vi "复材超声C扫缺陷分析评定软件.vi"() -> ()   [LabVIEW 2018]
doc: "使用该模板构建用户界面事件处理设计模式。将模板应用于对话框及其它用户界面。用户也可创建并执行VI可按照与用户界面事件相同方式处理的用户定义事件。"
uses:
  <vilib>/Utility/NIReport.llb/Report Type.ctl
  <vilib>/addons/_office/_exclsub.llb/font.ctl
  <vilib>/Utility/NIReport.llb/HTML Report Image Alignment.ctl
  <vilib>/Utility/NIReport.llb/Append Report Text (str wrap).vi
  <vilib>/Utility/NIReport.llb/Append Image to Report (path wrap).vi
  <vilib>/addons/_office/word.llb/Word Easy Table (str).vi
  <vilib>/Utility/NIReport.llb/NI_report.lvclass
  <vilib>/vision/NI_Vision_Development_Module.lvlib
  <vilib>/Utility/NIReport.llb/Word/NI_Word.lvclass
  <vilib>/addons/_office/NI_ReportGenerationToolkit.lvlib
  <vilib>/Utility/NIReport.llb/NI_ReportGenerationCore.lvlib
panel:
  in  "删除标注":bool caption="定量分析"
  out "输入的灰度阈值":dbl caption="值"
  out "反射图原始路径":path
  out "穿透图原始路径":path
  out "ROImask":T1(plugin-control)
  in  "Operation 2":enum16{"overlay rectangle"}(ring)
  out "模式选择":u16(ring) items=["只读穿透图", "穿透图和反射图结合"]
  out "添加的路径":path
  out "连接的字符串 2":string
  out "临界面积百分比值":dbl
  out "临界Z值":i32
  out "标注后的图片路径":path
  out "弥散类检测结果合并":string[][](table)
  out "分层类检测结果合并":string[][](table)
  out "弥散类检测结果":string[][](table)
  out "分层类检测结果":string[][](table)
  out "部位信息":string[](array[string])=["", "34.500000", "32.500000", "1121", "34", "54.955926", "分层类", "不合格", ""]
  out "连接的字符串":string
  in  "完成标注":bool caption="定量分析"
  out "框数":dbl
  in  "Operation":enum16{"overlay rectangle"}(ring)
  out "自定义字体":T2={"Desired Font (Application)"=enum."Application Font", "[User-specified Font]"={"Font Name"="", "Size"=12, "Strikeout?"=FALSE, "Italic?"=FALSE, "Underline?"=FALSE, "Outline?"=FALSE, "Shadow?"=FALSE, "Bold?"=FALSE, "Rotation Angle"=0.0}, "Horizontal Alignment"=0, "Vertical Alignment"=0} {"Horizontal Alignment" items=["Left", "Center", "Right"]; "Vertical Alignment" items=["Bottom", "Top", "Baseline"]}
  out "框组":T3(array[cluster])
  out "质量等级":string
  out "灰度阈值":dbl
  in  "stop":bool caption="停止"
  in  "导入图像":bool caption="导入图片"
  in  "图像预处理":bool
  in  "自定义色彩":bool
  in  "开始标注":bool caption="定量分析"
  in  "查看标注":bool caption="辅助定性分析"
  in  "生成评定结果":bool caption="生成原始记录"
  in  "?":enum32{"穿透图", "反射图"}(tab)
  out "穿透图":T1(plugin-control)
  out "反射图":T1(plugin-control)
  out "产品规格":cluster{"产品长度（周长）（mm）":dbl, "产品宽度（母线长）（mm）":dbl}
  out "图像分辨率":T4
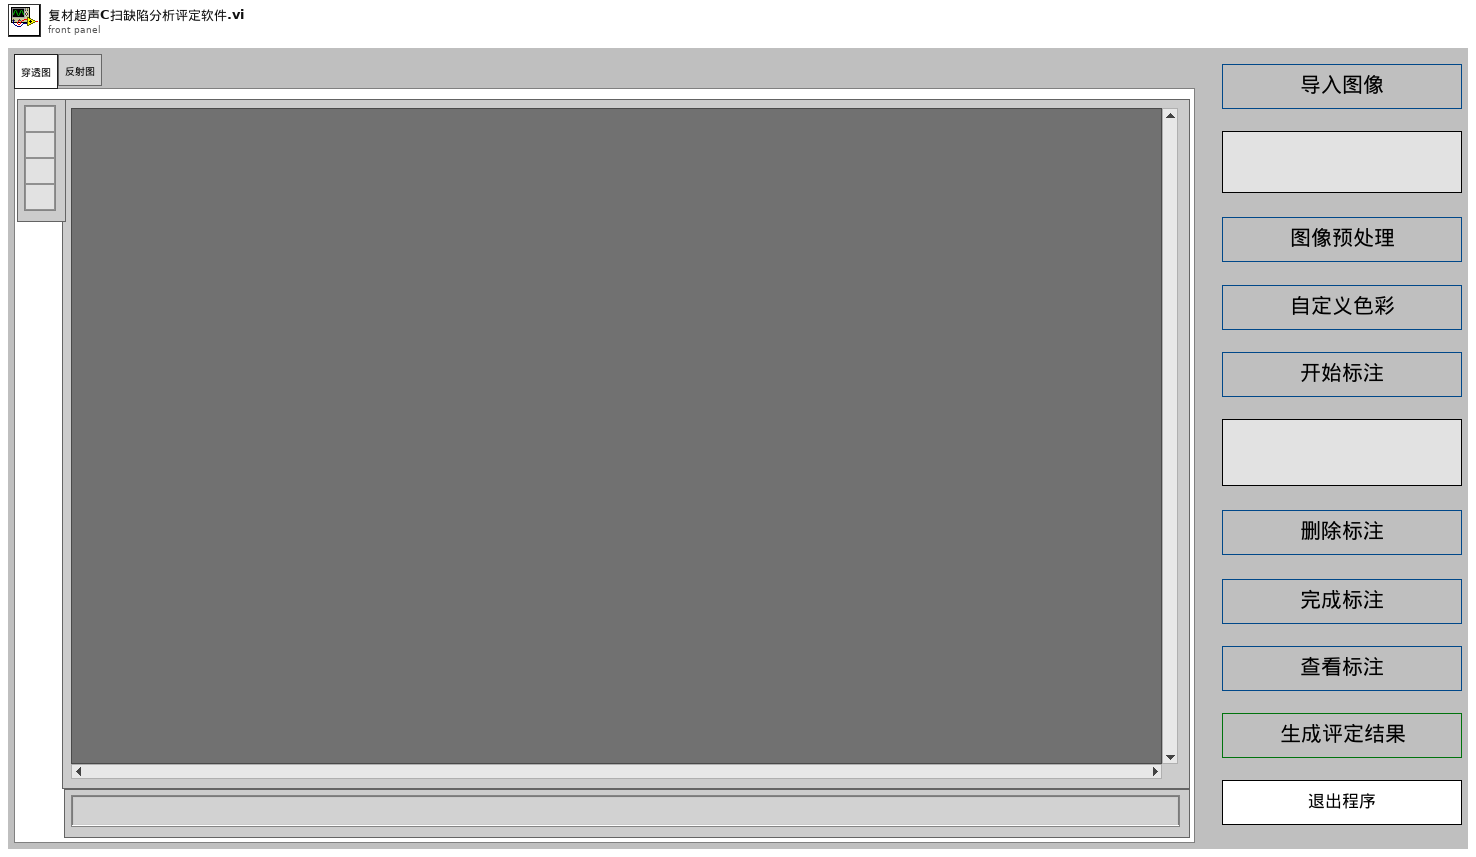
[diagram p1: front panel]
types:
  T1 = typedef "IMAQ Image.ctl" = refnum<image>
  T2 = cluster{"Desired Font (Application)":enum16{"User-specified Font", "Application Font", "System Font", "Dialog Font"}, "[User-specified Font]":cluster{"Font Name":string, "Size":i16, "Strikeout?":bool, "Italic?":bool, "Underline?":bool, "Outline?":bool, "Shadow?":bool, "Bold?":bool, "Rotation Angle":dbl}, "Horizontal Alignment":i16, "Vertical Alignment":i16}
  T3 = cluster{"Global Rectangle":i32[], "Contours":cluster{"Contour Type":u32, "ROI Type":u32, "Points":i32[]}[]}[]
  T4 = cluster{"图像X向分辨率（mm/像素）":dbl, "图像Y向分辨率（mm/像素）":dbl}
  T5 = cluster{"Zoom Tool":bool, "Selection Tool":bool, "Pan Tool":bool, "Point Tool":bool, "Line Tool":bool, "Rectangle Tool":bool, "Rotated Rectangle Tool":bool, "Polyline Tool":bool, "Polygon Tool":bool, "Freehand Tool":bool, "Closed Freehand Tool":bool, "Ellipse Tool":bool, "Annulus Tool":bool}
  T6 = enum32{"Invalid", "Standard", "Closed", "Hidden", "Minimized", "Maximized"}
  T7 = enum32{"Linear", "Log", "Exp", "Square", "Square root", "Power X", "Power 1/X"}
  T8 = enum32{"Gray", "Binary", "Gradient", "Rainbow", "Temperature"}
  T9 = enum16{"maximized", "minimized", "normal", "no change"}
  T10 = typedef "NI_ReportGenerationCore.lvlib/Report Type.ctl" = enum16{"HTML", "Word", "Excel"}
  T11 = typedef "NI_ReportGenerationCore.lvlib/HTML Report Image Alignment.ctl" = enum16{"(default)", "LEFT", "RIGHT", "TOP", "TEXTTOP", "MIDDLE", "ABSMIDDLE", "BASELINE", "BOTTOM", "ABSBOTTOM"}
  T12 = cluster{"position (Excel)":cluster{"row":i32, "column":i32}, "name (Excel)":string, "bookmark (Word)":string}
  T13 = cluster{"position (excel)":cluster{"row":i32, "column":i32}, "name (excel)":string, "bookmark (word)":string}
  T14 = typedef "NI_ReportGenerationToolkit.lvlib/font.ctl" = cluster{"font name":string, "font size":dbl, "bold":u16, "italic":u16, "underline":u16, "strike through":u16, "font color":u32}
  T15 = typedef "Image Type" = u32
  T16 = cluster{"Red (or Hue) value":u8, "Green (or Sat) value":u8, "Blue (or Light or Val) value":u8}[]
  T17 = cluster{"Global Rectangle":i32[], "Contours":cluster{"Contour Type":u32, "ROI Type":u32, "Points":i32[]}[]}
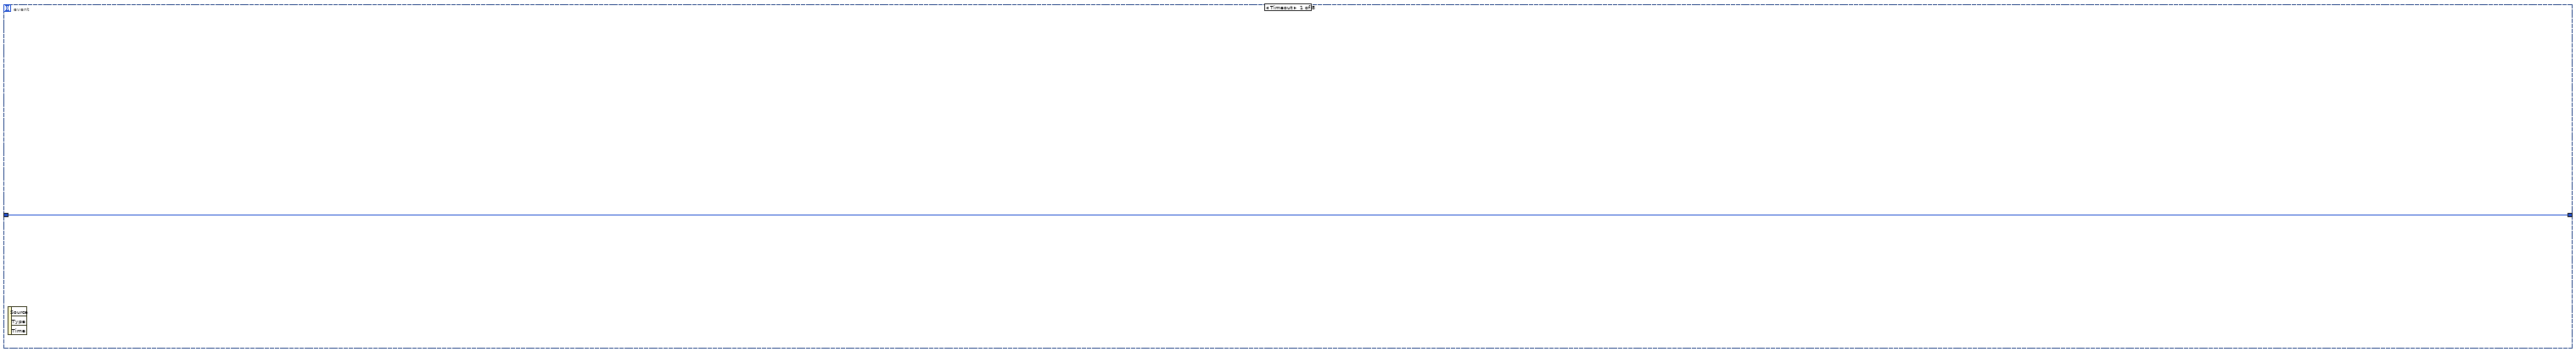
[diagram p3: hidden frame]
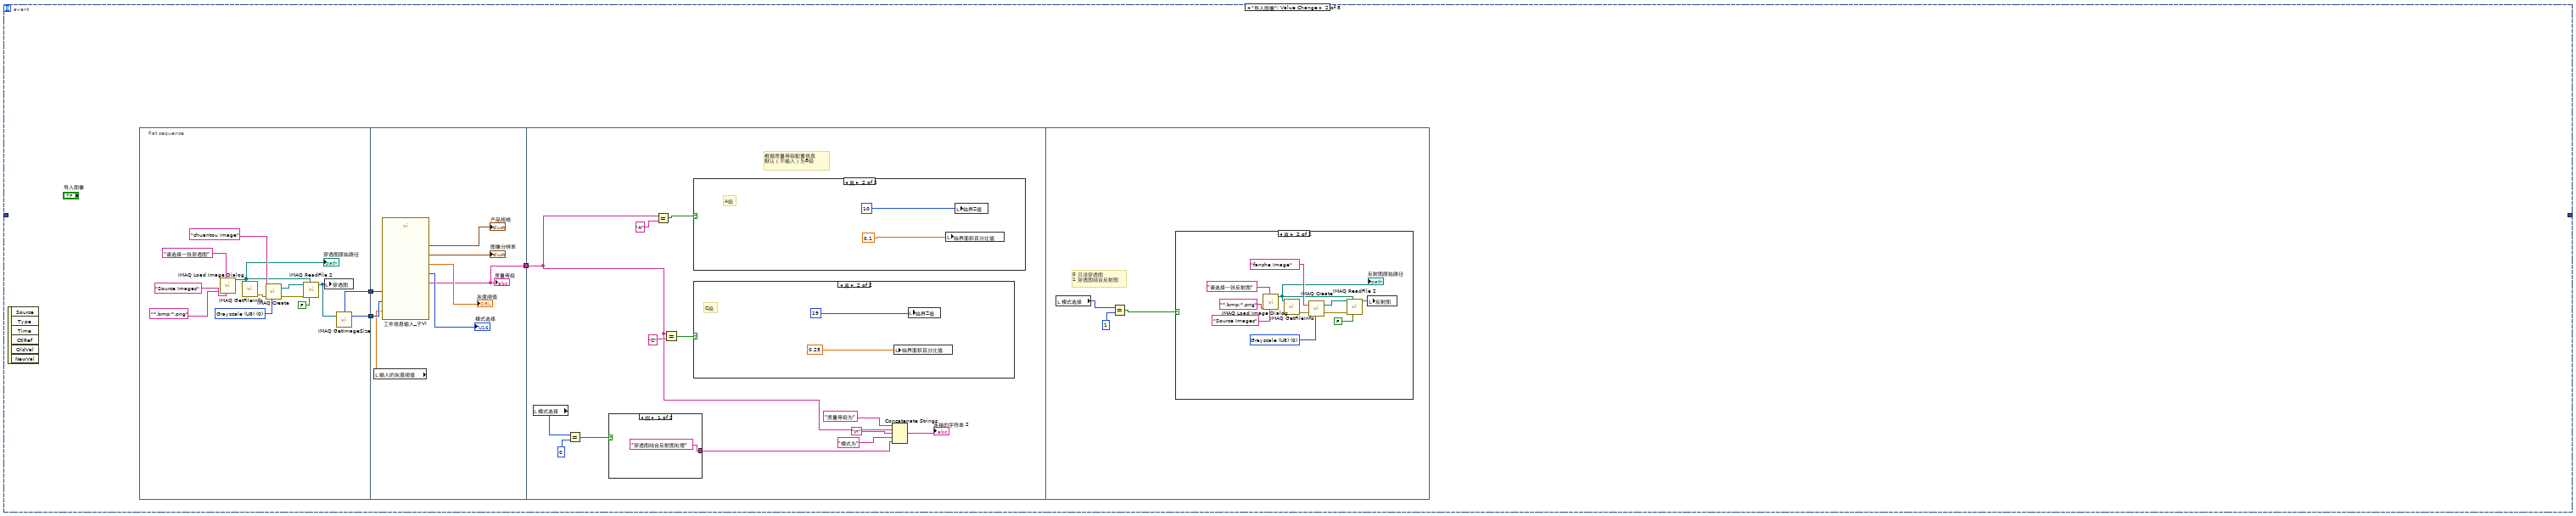
[diagram p4: hidden frame]
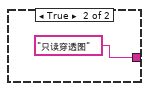
[diagram p5: hidden frame]
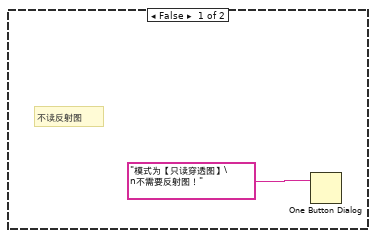
[diagram p8: hidden frame]
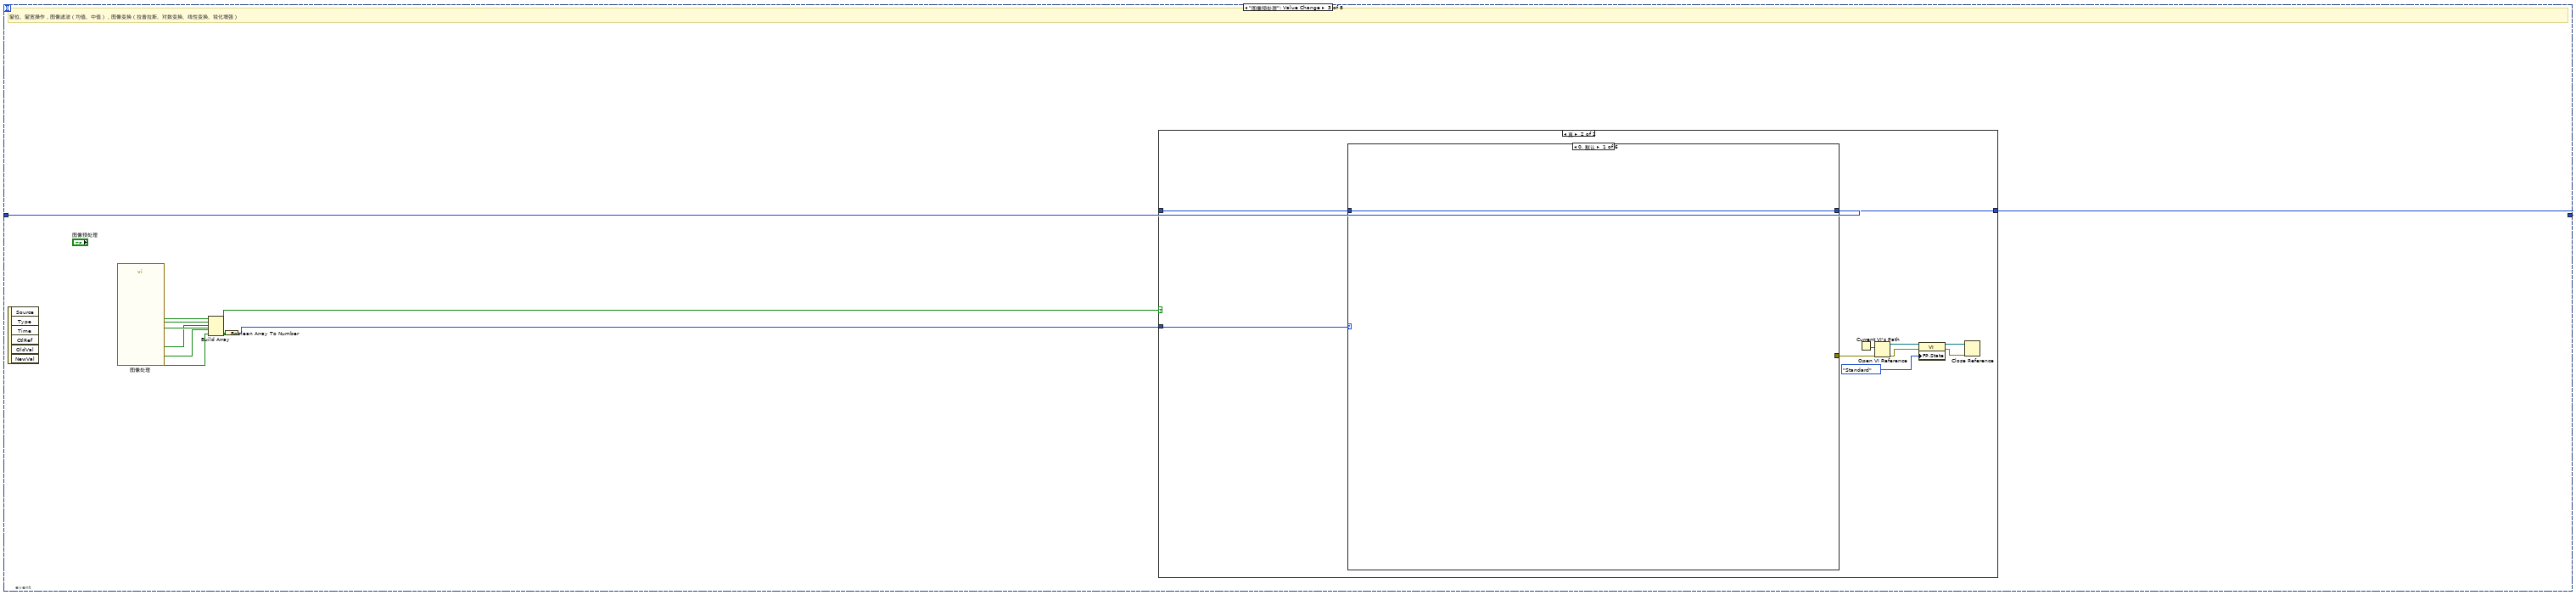
[diagram p9: hidden frame]
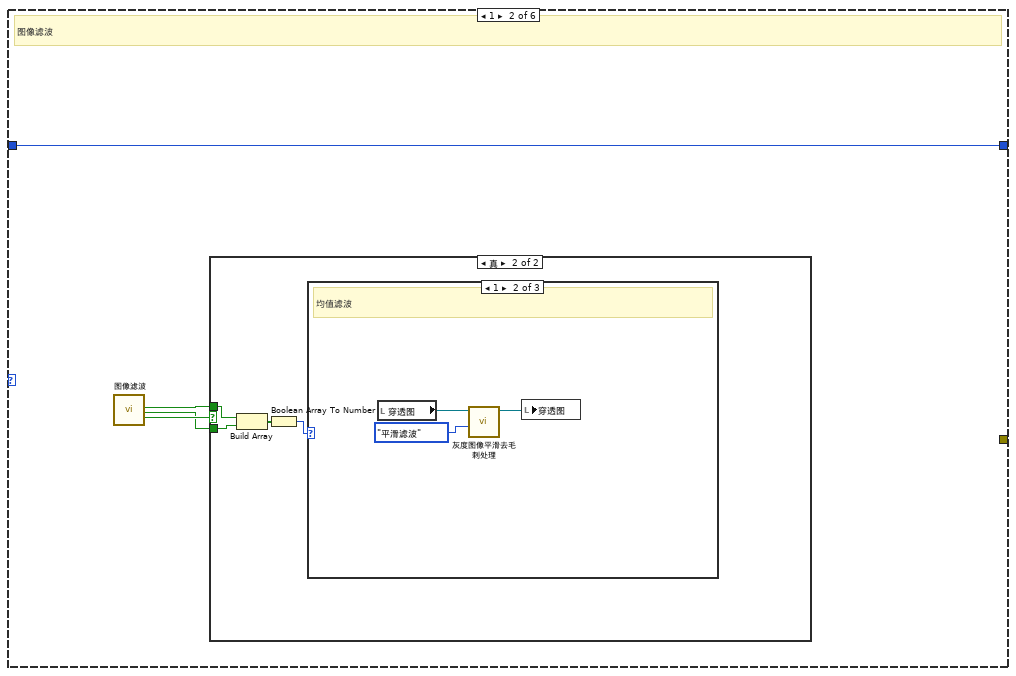
[diagram p11: hidden frame]
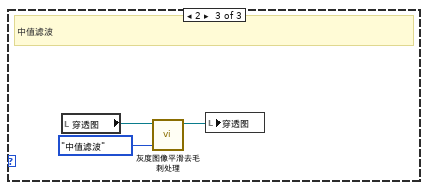
[diagram p14: hidden frame]
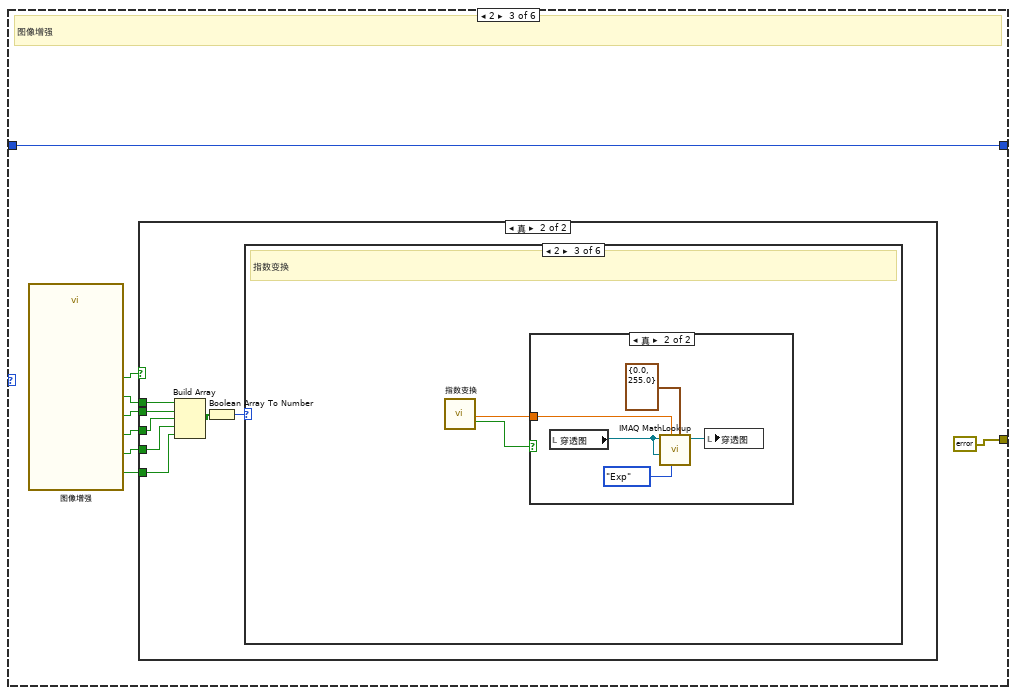
[diagram p15: hidden frame]
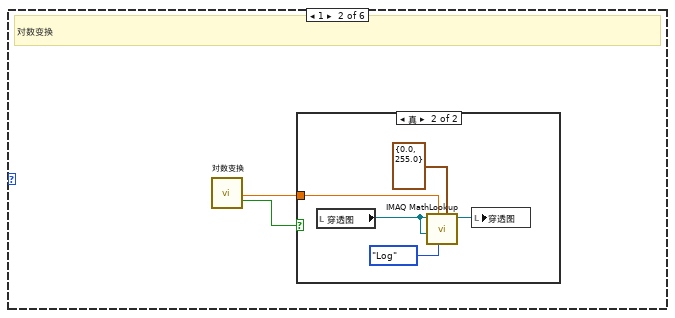
[diagram p18: hidden frame]
diagram:
  w12 = u16 0 items=["只读穿透图", "穿透图和反射图结合"] ("模式选择")
  w1 = FALSE ("查看标注")
  w17 = u32 0 items=["Grayscale", "Binary", "Gradient", "Rainbow", "Temperature", "User Defined", "Binary 16 Bit", "Gradient 16 Bit", "Rainbow 16 Bit", "Temperature 16 Bit", "User Defined 16 Bit"] ("Palette:Palette Type")
  w21 = TRUE ("Zoom to Fit Mode")
  w24 = u32 0 items=["Grayscale", "Binary", "Gradient", "Rainbow", "Temperature", "User Defined", "Binary 16 Bit", "Gradient 16 Bit", "Rainbow 16 Bit", "Temperature 16 Bit", "User Defined 16 Bit"] ("Palette:Palette Type")
  # "默认B级作为评判标准"
  n1 = flat-sequence {
    tunnel: [w28] -> w9
    tunnel: [w27] -> w8
    tunnel: [w26] -> w3
    tunnel: w9 -> [w31]
    tunnel: w8 -> [w32]
    tunnel: [w32] -> w7
    tunnel: [w31] -> w6
    tunnel: [w30] -> w4
    tunnel: w7 -> [w36]
    tunnel: w6 -> [w35]
    tunnel: [w34] -> w5
    frame #0 {
      w27 = "复材分析评定软件" ("section")
      w28 = "判定阈值配置" ("文件名称")
      n2 = call "ini配置文件读取（DBL）.vi"("key"="Z值", "section"=w27, "文件名称"=w28) -> ("value"=w26:dbl)  [unwired: 8 in]
    }
    frame #1 {
      n3 = call "ini配置文件读取（DBL）.vi"("key"="弥散性缺陷阈值", "section"=w32, "文件名称"=w31) -> ("value"=w30:dbl)  [unwired: 8 in]
    }
    frame #2 {
      n4 = call "ini配置文件读取（DBL）.vi"("key"="灰度阈值", "section"=w36, "文件名称"=w35) -> ("value"=w34:dbl)  [unwired: 8 in]
    }
  }
  n5 = To Long Integer(number=w3) -> (32bit integer=→"临界Z值":i32)
  n6 = property on="穿透图" class="ImageControl"("Palette Type"=w24, "ROI Tool Buttons Visible"=T5 {"Zoom Tool"=TRUE, "Selection Tool"=TRUE, "Pan Tool"=TRUE, "Point Tool"=FALSE, "Line Tool"=FALSE, "Rectangle Tool"=TRUE, "Rotated Rectangle Tool"=FALSE, "Polyline Tool"=FALSE, "Polygon Tool"=FALSE, "Freehand Tool"=FALSE, "Closed Freehand Tool"=FALSE, "Ellipse Tool"=FALSE, "Annulus Tool"=FALSE} ("ROI Tool Buttons Visible:All Elements")) -> ()  [unwired: 2 in, 2 out]
  n7 = property on="反射图" class="ImageControl"("Palette Type"=w17, "ROI Tool Buttons Visible"=T5 {"Zoom Tool"=TRUE, "Selection Tool"=TRUE, "Pan Tool"=TRUE, "Point Tool"=FALSE, "Line Tool"=FALSE, "Rectangle Tool"=TRUE, "Rotated Rectangle Tool"=FALSE, "Polyline Tool"=FALSE, "Polygon Tool"=FALSE, "Freehand Tool"=FALSE, "Closed Freehand Tool"=FALSE, "Ellipse Tool"=FALSE, "Annulus Tool"=FALSE} ("ROI Tool Buttons Visible:All Elements")) -> ()  [unwired: 2 in, 2 out]
  n8 = local write "标注后的图片路径"(path "" ("标注后的图片路径")) -> ()
  n9 = local write "连接的字符串 2"("（配置信息）" ("连接的字符串 2")) -> ()
  n10 = local write "连接的字符串"("（标注信息）" ("连接的字符串")) -> ()
  n11 = property on="穿透图" class="ImageControl"("Zoom to Fit Mode"=w21) -> ()  [unwired: 2 in, 2 out]
  n12 = property on="反射图" class="ImageControl"("Zoom to Fit Mode"=w21) -> ()  [unwired: 2 in, 2 out]
  n13 = local write "删除标注"(w1) -> ()
  n14 = local write "查看标注"(w1) -> ()
  n15 = local write "模式选择"(w12) -> ()
  n16 = local write "stop"(w1) -> ()
  n17 = local write "完成标注"(w1) -> ()
  n18 = while {
    shift-right: [w38] -> _
    shift-left: 0 -> [w39]
    stop <- w41 stop-if-true
    n19 = event shown="[4] \"开始标注\": 鼠标按下" {
      selector: _ -> [_ _ _ _ _ _ _ _]
      dyn-events: _ -> [_ _ _ _ _ _ _ _]
      timeout: 100 -> [_ _ _ _ _ _ _ _]
      tunnel: [_ _ _ _ _ _ _ w756] -> w41
      tunnel: w39 -> [w42 _ w102 w240 _ _ w595 _]
      tunnel: [w42 _ w101 w240 _ _ w595 0] -> w38
      event Timeout {
        n20 = event-data() -> ()  [unwired: 1 in, 3 out]
      }
      event "导入图像": Value Change {
        n21 = event-data() -> ()  [unwired: 1 in, 6 out]
        n22 = flat-sequence {
          tunnel: [w47] -> w44
          tunnel: [w46] -> w43
          tunnel: [w62] -> w45
          tunnel: w44 -> [w61]
          tunnel: w43 -> [w60]
          tunnel: w45 -> [w71]
          frame #0 {
            w50 = T15 0 items=["Grayscale (U8)", "Grayscale (I16)", "Grayscale (SGL)", "Complex (CSG)", "RGB (U32)", "HSL (U32)", "RGB (U64)", "Grayscale (U16)"] ("Image Type")
            n23 = call "IMAQ Load Image Dialog"("Pattern Label"="Source Images", "Prompt"="请选择一张穿透图" ("prompt"), "Pattern"="*.bmp;*.png") -> ("Path"=w49:path)  [unwired: 6 in, 2 out]
            "穿透图原始路径" <- w49
            n24 = call "IMAQ GetFileInfo"("File Path"=w49) -> ("error out"=w53:errorcluster)  [unwired: 4 in, 6 out]
            n25 = call "IMAQ Create"("Image Name"="chuantou Image", "Image Type"=w50, "error in (no error)"=w53) -> ("New Image"=w54:T1, "error out"=w55:errorcluster)  [unwired: 2 in]
            n26 = call "IMAQ ReadFile 2"("Use File Path Image Type"=FALSE, "File Path"=w49, "error in (no error)"=w55, "Image"=w54) -> ("Image Out"=w48:T1)  [unwired: 3 in, 4 out]
            n27 = local write "穿透图"(w48) -> ()
            n28 = call "IMAQ GetImageSize"("Image"=w48) -> ("Y Resolution"=w46:i32, "X Resolution"=w47:i32)  [unwired: 3 in, 1 out]
          }
          frame #1 {
            n29 = local read "输入的灰度阈值"() -> (w59:dbl)
            n30 = call "工件信息输入_子VI.vi"("Y Resolution"=w60, "X Resolution"=w61, "输入的灰度阈值"=w59) -> ("质量等级"=w62:string, "模式选择"=→"模式选择":u16, "灰度阈值"=→"灰度阈值":dbl, "产品规格"=→"产品规格":cluster{"产品长度（周长）（mm）":dbl, "产品宽度（母线长）（mm）":dbl}, "图像分辨率"=→"图像分辨率":T4)  [unwired: 3 in]
            "质量等级" <- w62
          }
          frame #2 {
            # "根据质量等级配置信息\n默认（不输入）为B级"
            n31 = local read "模式选择"() -> (w69:u16)
            n32 = Equal?(x=w69, y=u16 0) -> (x = y?=w68:bool)
            n33 = case shown="假" w68 {
              tunnel: ["穿透图结合反射图处理" ("字符串") "只读穿透图" ("字符串")] -> w67
              frame False {
              }
              frame True {
              }
            }
            n34 = Equal?(x=w71, y="A") -> (x = y?=w74:bool)
            n35 = Equal?(x=w71, y="C") -> (x = y?=w75:bool)
            n36 = case shown="真" w74 {
              frame False {
              }
              frame True {
                # "A级"
                n37 = local write "临界面积百分比值"(0.1 ("临界面积百分比值")) -> ()
                n38 = local write "临界Z值"(10 ("临界Z值")) -> ()
              }
            }
            n39 = case shown="真" w75 {
              frame False {
              }
              frame True {
                # "C级"
                n40 = local write "临界面积百分比值"(0.25 ("临界面积百分比值")) -> ()
                n41 = local write "临界Z值"(19 ("临界Z值")) -> ()
              }
            }
            n42 = Concatenate Strings("质量等级为" ("字符串"), w71, "\n", "模式为" ("字符串"), w67) -> (→"连接的字符串 2":string)
          }
          frame #3 {
            # "0 只读穿透图\n1 穿透图结合反射图"
            n43 = local read "模式选择"() -> (w87:u16)
            n44 = Equal?(x=w87, y=u16 1) -> (x = y?=w86:bool)
            n45 = case shown="真" w86 {
              frame False {
                # "不读反射图"
                n46 = One Button Dialog(message="模式为【只读穿透图】\n不需要反射图！" ("消息")) -> ()  [unwired: 1 in, 1 out]
              }
              frame True {
                w92 = T15 0 items=["Grayscale (U8)", "Grayscale (I16)", "Grayscale (SGL)", "Complex (CSG)", "RGB (U32)", "HSL (U32)", "RGB (U64)", "Grayscale (U16)"] ("Image Type")
                n47 = call "IMAQ Load Image Dialog"("Pattern Label"="Source Images", "Prompt"="请选择一张反射图" ("prompt"), "Pattern"="*.bmp;*.png") -> ("Path"=w91:path)  [unwired: 6 in, 2 out]
                "反射图原始路径" <- w91
                n48 = call "IMAQ GetFileInfo"("File Path"=w91) -> ("error out"=w95:errorcluster)  [unwired: 4 in, 6 out]
                n49 = call "IMAQ Create"("Image Name"="fanshe Image", "Image Type"=w92, "error in (no error)"=w95) -> ("New Image"=w96:T1, "error out"=w97:errorcluster)  [unwired: 2 in]
                n50 = call "IMAQ ReadFile 2"("Use File Path Image Type"=FALSE, "File Path"=w91, "error in (no error)"=w97, "Image"=w96) -> ("Image Out"=w90:T1)  [unwired: 3 in, 4 out]
                n51 = local write "反射图"(w90) -> ()
              }
            }
          }
        }
      }
      event "图像预处理": Value Change {
        # "窗位、窗宽操作，图像滤波（均值、中值），图像变换（拉普拉斯、对数变换、线性变换、锐化增强）"
        n52 = event-data() -> ()  [unwired: 1 in, 6 out]
        n53 = call "图像处理"() -> ("撤销图像处理"=w103:bool, "线性灰度值测量"=w104:bool, "窗位窗宽"=w109:bool, "图像增强"=w105:bool, "图像滤波"=w110:bool, "确定"=w106:bool)  [unwired: 13 in, 1 out]
        n54 = Build Array(w110, w105, w109, w104, w103) -> (w108:bool[])
        n55 = Boolean Array To Number(Boolean array=w108) -> (number=w107:u32)
        n56 = case shown="真" w106 {
          tunnel: w107 -> [_ w121]
          tunnel: w102 -> [w111 w113]
          tunnel: [w111 w112] -> w101
          frame False {
          }
          frame True {
            n57 = case shown="0, 默认" w121 {
              tunnel: [_ _ errorcluster {"status"=FALSE, "code"=0, "source"=""} ("错误输入（无错误）") _ _ _] -> w114
              tunnel: w113 -> [w122 w123 w137 w186 w209 w231]
              tunnel: [w122 w123 w137 w186 w209 w231] -> w112
              frame 0, Default {
              }
              frame 1 {
                # "图像滤波"
                n58 = call "图像滤波"() -> ("均值滤波"=w125:bool, "中值滤波"=w124:bool, "确定"=w126:bool)  [unwired: 16 in, 1 out]
                n59 = case shown="真" w126 {
                  tunnel: w125 -> [_ w129]
                  tunnel: w124 -> [_ w128]
                  frame False {
                  }
                  frame True {
                    n60 = Build Array(w129, w128) -> (w130:bool[])
                    n61 = Boolean Array To Number(Boolean array=w130) -> (number=w127:u32)
                    n62 = case shown="1" w127 {
                      frame 0, Default {
                      }
                      frame 1 {
                        # "均值滤波"
                        n63 = local read "穿透图"() -> (w133:T1)
                        n64 = call "灰度图像平滑去毛刺处理.vi"("滤波方法选择"=enum16{"中值滤波", "平滑滤波"}."平滑滤波", "Image"=w133) -> ("Image Out"=w132:T1)  [unwired: 9 in]
                        n65 = local write "穿透图"(w132) -> ()
                      }
                      frame 2 {
                        # "中值滤波"
                        n66 = local read "穿透图"() -> (w136:T1)
                        n67 = call "灰度图像平滑去毛刺处理.vi"("滤波方法选择"=enum16{"中值滤波", "平滑滤波"}."中值滤波", "Image"=w136) -> ("Image Out"=w135:T1)  [unwired: 9 in]
                        n68 = local write "穿透图"(w135) -> ()
                      }
                    }
                  }
                }
              }
              frame 2 {
                # "图像增强"
                n69 = call "图像增强"() -> ("幂变换"=w139:bool, "阈值变换"=w140:bool, "高斯变换"=w141:bool, "指数变换"=w142:bool, "对数变换"=w143:bool, "确定"=w144:bool)  [unwired: 13 in, 1 out]
                n70 = case shown="真" w144 {
                  tunnel: w143 -> [_ w149]
                  tunnel: w142 -> [_ w148]
                  tunnel: w141 -> [_ w147]
                  tunnel: w140 -> [_ w146]
                  tunnel: w139 -> [_ w145]
                  frame False {
                  }
                  frame True {
                    n71 = Build Array(w149, w148, w147, w146, w145) -> (w151:bool[])
                    n72 = Boolean Array To Number(Boolean array=w151) -> (number=w150:u32)
                    n73 = case shown="2" w150 {
                      frame 0, Default {
                      }
                      frame 1 {
                        # "对数变换"
                        n74 = call "对数变换"() -> ("变换系数K"=w152:dbl, "确定"=w153:bool)  [unwired: 17 in, 1 out]
                        n75 = case shown="真" w153 {
                          tunnel: w152 -> [_ w154]
                          frame False {
                          }
                          frame True {
                            n76 = local read "穿透图"() -> (w158:T1)
                            n77 = call "IMAQ MathLookup"("Range"=cluster{"Minimum":sgl, "Maximum":sgl} {"Minimum"=0.0, "Maximum"=255.0}, "Operator"=T7."Log", "X Value"=w154, "Image Dst"=w158, "Image Src"=w158) -> ("Image Dst Out"=w156:T1)  [unwired: 5 in, 1 out]
                            n78 = local write "穿透图"(w156) -> ()
                          }
                        }
                      }
                      frame 2 {
                        # "指数变换"
                        n79 = call "指数变换"() -> ("变换系数K"=w159:dbl, "确定"=w160:bool)  [unwired: 17 in, 1 out]
                        n80 = case shown="真" w160 {
                          tunnel: w159 -> [_ w161]
                          frame False {
                          }
                          frame True {
                            n81 = local read "穿透图"() -> (w165:T1)
                            n82 = call "IMAQ MathLookup"("Range"=cluster{"Minimum":sgl, "Maximum":sgl} {"Minimum"=0.0, "Maximum"=255.0}, "Operator"=T7."Exp", "X Value"=w161, "Image Dst"=w165, "Image Src"=w165) -> ("Image Dst Out"=w163:T1)  [unwired: 5 in, 1 out]
                            n83 = local write "穿透图"(w163) -> ()
                          }
                        }
                      }
                      frame 4 {
                        w171 = u16 4 items=["Gradient"=1, "Laplacian"=2, "Smoothing"=3, "Gaussian"=4] ("Kernel Family")
                        # "高斯斯变换"
                        n84 = local read "穿透图"() -> (w168:T1)
                        n85 = call "IMAQ GetKernel"("Kernel Family"=w171, "Kernel Size (3,5,...)"=3) -> ("Kernel"=w169:sgl[][], "Divider"=w166:sgl)  [unwired: 6 in, 2 out]
                        n86 = call "IMAQ Convolute"("Kernel"=w169, "Divider (kernel sum)"=w166, "Image Dst"=w168, "Image Src"=w168) -> ("Image Dst Out"=w167:T1)  [unwired: 6 in, 1 out]
                        n87 = local write "穿透图"(w167) -> ()
                      }
                      frame 8 {
                        # "阈值变换"
                        n88 = call "阈值范围选择子VI.vi"() -> ("阈值范围"=w172:cluster{"Lower value":sgl, "Upper value":sgl}, "确定执行"=w173:bool)  [unwired: 10 in]
                        n89 = case shown="真" w173 {
                          tunnel: w172 -> [_ w175]
                          frame False {
                          }
                          frame True {
                            n90 = local read "穿透图"() -> (w178:T1)
                            n91 = call "IMAQ Threshold"("Replace Value"=sgl 255.0, "Keep/Replace Value (Replace)"=TRUE, "Range"=w175, "Image Dst"=w178, "Image Src"=w178) -> ("Image Dst Out"=w177:T1)  [unwired: 5 in, 1 out]
                            n92 = local write "穿透图"(w177) -> ()
                          }
                        }
                      }
                      frame 16 {
                        # "幂变换"
                        n93 = call "幂变换"() -> ("变换系数K"=w179:dbl, "确定"=w180:bool)  [unwired: 17 in, 1 out]
                        n94 = case shown="真" w180 {
                          tunnel: w179 -> [_ w181]
                          frame False {
                          }
                          frame True {
                            n95 = local read "穿透图"() -> (w185:T1)
                            n96 = call "IMAQ MathLookup"("Range"=cluster{"Minimum":sgl, "Maximum":sgl} {"Minimum"=0.0, "Maximum"=255.0}, "Operator"=T7."Power 1/X", "X Value"=w181, "Image Dst"=w185, "Image Src"=w185) -> ("Image Dst Out"=w183:T1)  [unwired: 5 in, 1 out]
                            n97 = local write "穿透图"(w183) -> ()
                          }
                        }
                      }
                    }
                  }
                }
              }
              frame 4 {
                # "窗位窗宽"
                n98 = Two Button Dialog(message="确定进行窗位窗宽操作？" ("消息")) -> (T button?=w188:bool)  [unwired: 2 in]
                n99 = case shown="真" w188 {
                  frame False {
                  }
                  frame True {
                    n100 = property on="穿透图" class="ImageControl"() -> (error out=w190:errorcluster, "Palette Type"=w197:u32)  [unwired: 2 in, 1 out]
                    n101 = Current VI's Path() -> (path=w192:path)
                    n102 = Open VI Reference(vi path=w192, error in (no error)=w190) -> (vi reference=w193:refnum<vi>, error out=w195:errorcluster)  [unwired: 4 in]
                    n103 = case shown="4" w197 {
                      tunnel: [w200 w202 w204 w206 w208] -> w198
                      frame 0, Default {
                        # "灰度"
                        n104 = call "IMAQ GetPalette"("Palette Number (gray)"=T8."Gray") -> ("Color Palette"=w200:cluster{"Red":u8, "Green":u8, "Blue":u8}[])  [unwired: 4 in, 1 out]
                      }
                      frame 2 {
                        # "梯度"
                        n105 = call "IMAQ GetPalette"("Palette Number (gray)"=T8."Gradient") -> ("Color Palette"=w202:cluster{"Red":u8, "Green":u8, "Blue":u8}[])  [unwired: 4 in, 1 out]
                      }
                      frame 3 {
                        # "彩虹"
                        n106 = call "IMAQ GetPalette"("Palette Number (gray)"=T8."Rainbow") -> ("Color Palette"=w204:cluster{"Red":u8, "Green":u8, "Blue":u8}[])  [unwired: 4 in, 1 out]
                      }
                      frame 4 {
                        # "温度"
                        n107 = call "IMAQ GetPalette"("Palette Number (gray)"=T8."Temperature") -> ("Color Palette"=w206:cluster{"Red":u8, "Green":u8, "Blue":u8}[])  [unwired: 4 in, 1 out]
                      }
                      frame 5 {
                        # "自定义"
                        n108 = property on="穿透图" class="ImageControl"() -> ("User Palette"=w208:cluster{"Red":u8, "Green":u8, "Blue":u8}[])  [unwired: 2 in, 2 out]
                      }
                    }
                    n109 = property class="VI"(reference=w193, error in=w195, "FP.State"=T6."Hidden" ("前面板窗口:状态")) -> (reference out=w194:refnum<vi>, error out=w196:errorcluster)
                    n110 = Close Reference(reference=w194, error in (no error)=w196) -> ()  [unwired: 1 out]
                    n111 = local read "穿透图"() -> (w189:T1)
                    n112 = call "窗位窗宽调整子VI.vi"("Image in"=w189, "Palette:User Palette"=w198, "Palette:Palette Type"=w197) -> ("Image out"=w199:T1)  [unwired: 8 in]
                    n113 = local write "穿透图"(w199) -> ()
                  }
                }
              }
              frame 8 {
                # "查看线灰度值曲线，用于精确测量"
                n114 = Current VI's Path() -> (path=w216:path)
                n115 = Open VI Reference(vi path=w216) -> (vi reference=w215:refnum<vi>, error out=w213:errorcluster)  [unwired: 5 in]
                n116 = property class="VI"(reference=w215, error in=w213, "FP.State"=T6."Hidden" ("前面板窗口:状态")) -> (reference out=w214:refnum<vi>, error out=w212:errorcluster)
                n117 = Close Reference(reference=w214, error in (no error)=w212) -> (error out=w210:errorcluster)
                n118 = case shown="无错误" w210 {
                  frame No Error {
                    n119 = property on="穿透图" class="ImageControl"() -> ("Palette Type"=w218:u32)  [unwired: 2 in, 2 out]
                    n120 = case shown="2" w218 {
                      tunnel: [w221 w223 w225 w227 w229] -> w217
                      frame 0, Default {
                        # "灰度"
                        n121 = call "IMAQ GetPalette"("Palette Number (gray)"=T8."Gray") -> ("Color Palette"=w221:cluster{"Red":u8, "Green":u8, "Blue":u8}[])  [unwired: 4 in, 1 out]
                      }
                      frame 2 {
                        # "梯度"
                        n122 = call "IMAQ GetPalette"("Palette Number (gray)"=T8."Gradient") -> ("Color Palette"=w223:cluster{"Red":u8, "Green":u8, "Blue":u8}[])  [unwired: 4 in, 1 out]
                      }
                      frame 3 {
                        # "彩虹"
                        n123 = call "IMAQ GetPalette"("Palette Number (gray)"=T8."Rainbow") -> ("Color Palette"=w225:cluster{"Red":u8, "Green":u8, "Blue":u8}[])  [unwired: 4 in, 1 out]
                      }
                      frame 4 {
                        # "温度"
                        n124 = call "IMAQ GetPalette"("Palette Number (gray)"=T8."Temperature") -> ("Color Palette"=w227:cluster{"Red":u8, "Green":u8, "Blue":u8}[])  [unwired: 4 in, 1 out]
                      }
                      frame 5 {
                        # "自定义"
                        n125 = property on="穿透图" class="ImageControl"() -> ("User Palette"=w229:cluster{"Red":u8, "Green":u8, "Blue":u8}[])  [unwired: 2 in, 2 out]
                      }
                    }
                    n126 = local read "穿透图"() -> (w220:T1)
                    n127 = local read "图像分辨率"() -> (w219:T4)
                    n128 = call "线性灰度值曲线查看子VI.vi"("Palette:User Palette"=w217, "图像分辨率"=w219, "Image"=w220) -> ()  [unwired: 9 in]
                  }
                  frame Error {
                  }
                }
              }
              frame 16 {
                # "撤销图像处理，恢复原图"
                n129 = call "IMAQ Create"("Image Name"="P1") -> ("New Image"=w230:T1)  [unwired: 4 in, 1 out]
                n130 = local write "穿透图"(w230) -> ()
              }
            }
            n131 = Current VI's Path() -> (path=w120:path)
            n132 = Open VI Reference(vi path=w120, error in (no error)=w114) -> (vi reference=w119:refnum<vi>, error out=w116:errorcluster)  [unwired: 4 in]
            n133 = property class="VI"(reference=w119, error in=w116, "FP.State"=T6."Standard" ("前面板窗口:状态")) -> (reference out=w117:refnum<vi>, error out=w115:errorcluster)
            n134 = Close Reference(reference=w117, error in (no error)=w115) -> ()  [unwired: 1 out]
          }
        }
      }
      event "自定义色彩": Value Change {
        # "色彩、色阶自定义"
        n135 = event-data() -> ()  [unwired: 1 in, 6 out]
        n136 = call "调色板"() -> ("自定义显示"=w234:bool, "温度显示"=w235:bool, "彩虹显示"=w236:bool, "梯度显示"=w237:bool, "灰度显示"=w238:bool, "确定"=w239:bool)  [unwired: 13 in, 1 out]
        n137 = Build Array(w238, w237, w236, w235, w234) -> (w233:bool[])
        n138 = case shown="真" w239 {
          tunnel: w233 -> [_ w243]
          frame False {
          }
          frame True {
            n139 = Boolean Array To Number(Boolean array=w243) -> (number=w242:u32)
            n140 = case shown="0, 默认" w242 {
              tunnel: [w244 w245 w246 w247 w248 w250] -> w241
              frame 0, Default {
                w244 = u32 0 items=["Grayscale", "Binary", "Gradient", "Rainbow", "Temperature", "User Defined", "Binary 16 Bit", "Gradient 16 Bit", "Rainbow 16 Bit", "Temperature 16 Bit", "User Defined 16 Bit"] ("Palette:Palette Type")
              }
              frame 1 {
                w245 = u32 0 items=["Grayscale", "Binary", "Gradient", "Rainbow", "Temperature", "User Defined", "Binary 16 Bit", "Gradient 16 Bit", "Rainbow 16 Bit", "Temperature 16 Bit", "User Defined 16 Bit"] ("Palette:Palette Type")
                # "灰度"
              }
              frame 2 {
                w246 = u32 2 items=["Grayscale", "Binary", "Gradient", "Rainbow", "Temperature", "User Defined", "Binary 16 Bit", "Gradient 16 Bit", "Rainbow 16 Bit", "Temperature 16 Bit", "User Defined 16 Bit"] ("Palette:Palette Type")
                # "梯度"
              }
              frame 4 {
                w247 = u32 3 items=["Grayscale", "Binary", "Gradient", "Rainbow", "Temperature", "User Defined", "Binary 16 Bit", "Gradient 16 Bit", "Rainbow 16 Bit", "Temperature 16 Bit", "User Defined 16 Bit"] ("Palette:Palette Type")
                # "彩虹"
              }
              frame 8 {
                w248 = u32 4 items=["Grayscale", "Binary", "Gradient", "Rainbow", "Temperature", "User Defined", "Binary 16 Bit", "Gradient 16 Bit", "Rainbow 16 Bit", "Temperature 16 Bit", "User Defined 16 Bit"] ("Palette:Palette Type")
                # "温度"
              }
              frame 16 {
                w250 = u32 5 items=["Grayscale", "Binary", "Gradient", "Rainbow", "Temperature", "User Defined", "Binary 16 Bit", "Gradient 16 Bit", "Rainbow 16 Bit", "Temperature 16 Bit", "User Defined 16 Bit"] ("Palette:Palette Type")
                # "自定义"
                n141 = call "自定义成像色谱20200214.vi"() -> ("Color palette"=w249:T16)  [unwired: 8 in, 1 out]
                n142 = property on="穿透图" class="ImageControl"("User Palette"=w249) -> ()  [unwired: 2 in, 2 out]
              }
            }
            n143 = property on="穿透图" class="ImageControl"("Palette Type"=w241) -> ()  [unwired: 2 in, 2 out]
          }
        }
      }
      event "开始标注": Mouse Down {
        w251 = FALSE ("完成标注")
        # "0 只读穿透图\n1 穿透图和反射图结合"
        # "手动画框ROI，提取框组（坐标）、框数等信息"
        n144 = event-data() -> ()  [unwired: 1 in, 6 out]
        n145 = local read "模式选择"() -> (w252:u16)
        n146 = One Button Dialog(message="开始标注！\n全部标注完成后，\n请点击“完成标注”按钮" ("消息")) -> ()  [unwired: 1 in, 1 out]
        n147 = local write "删除标注"(w251) -> ()
        n148 = local write "完成标注"(w251) -> ()
        n149 = local write "查看标注"(w251) -> ()
        n150 = case shown="0, 默认" w252 {
          tunnel: w251 -> [_ _]
          frame 0, Default {
            # "只对穿透图时画框的分支"
            n151 = while {
              shift-right: [w266] -> _
              shift-left: _ -> [w265]
              tunnel: [w263] -> _
              stop <- w256 stop-if-true
              (unwired) "_" ("名称或相对路径")
              (unwired) ".docx" ("名称或相对路径")
              w261 = i32[] [2] items=["No Event"=0, "Click Event"=1, "Draw Event"=2, "Size Event"=4, "Scroll Event"=5, "Double Click Event"=8] ("Which Events")
              # "循环的方式给输入图像手动画框"
              n152 = local read "穿透图"() -> (w264:T1)
              n153 = invoke on="穿透图" class="ImageControl" method="Get Last Event"("Which Events"=w261) -> ("Type"=w255:i32)  [unwired: 7 in, 7 out]
              n154 = property on="穿透图" class="ImageControl"() -> ("ROI"=w258:T17)  [unwired: 2 in, 2 out]
              n155 = Not Equal To 0?(x=w255) -> (x != 0?=w254:bool)
              n156 = case shown="真" w254 {
                tunnel: w264 -> [w275 w319]
                tunnel: [w275 w318] -> w263
                tunnel: "Operation 2" -> [_ w317]
                tunnel: [w273 w315] -> w266
                tunnel: w265 -> [w273 w316]
                tunnel: w258 -> [_ w314]
                frame False {
                  n157 = event shown="[1] \"查看标注\": 鼠标按下" {
                    selector: _ -> [_ _]
                    dyn-events: _ -> [_ _]
                    timeout: 50 -> [_ _]
                    event Timeout {
                      n158 = event-data() -> ()  [unwired: 1 in, 3 out]
                    }
                    event "查看标注": Mouse Down {
                      n159 = event-data() -> ()  [unwired: 1 in, 8 out]
                      n160 = local read "穿透图原始路径"() -> (w280:path)
                      n161 = local read "临界面积百分比值"() -> (w277:dbl)
                      n162 = local read "部位信息"() -> (w282:string[])
                      n163 = local read "临界Z值"() -> (w278:i32)
                      n164 = local read "产品规格"() -> (w281:cluster{"产品长度（周长）（mm）":dbl, "产品宽度（母线长）（mm）":dbl})
                      n165 = local read "灰度阈值"() -> (w276:dbl)
                      n166 = local read "框组"() -> (w279:T3)
                      n167 = call "输入选择框号"() -> ("框号"=w283:dbl)  [unwired: 17 in, 2 out]
                      n168 = call "子界面-查看某框-只读穿透图模式.vi"("框号"=w283, "框组"=w279, "临界Z值"=w278, "临界面积百分比值"=w277, "预先配置的灰度阈值"=w276, "穿透图原始路径"=w280, "部位信息"=w282, "产品规格"=w281) -> ()  [unwired: 10 in, 2 out]
                    }
                  }
                  n169 = Wait (ms)(milliseconds to wait=u32 100 ("毫秒倍数")) -> ()  [unwired: 1 out]
                  n170 = event shown="[1] \"删除标注\": 鼠标按下" {
                    selector: _ -> [_ _]
                    dyn-events: _ -> [_ _]
                    timeout: 50 -> [_ _]
                    event Timeout {
                      n171 = event-data() -> ()  [unwired: 1 in, 3 out]
                    }
                    event "删除标注": Mouse Down {
                      n172 = event-data() -> ()  [unwired: 1 in, 3 out]
                      n173 = call "用户输入2"() -> ("框号"=w284:dbl, "确定"=w285:bool)  [unwired: 17 in, 1 out]
                      n174 = case shown="真" w285 {
                        tunnel: w284 -> [_ w286]
                        frame False {
                          # "用户取消操作"
                        }
                        frame True {
                          n175 = stacked-sequence {
                            tunnel: w286 -> [_ w293 _]
                            frame #0 {
                              # "1. 删除所有框"
                              n176 = local read "穿透图"() -> (w287:T1)
                              n177 = call "IMAQ Clear Overlay"("Image"=w287) -> ()  [unwired: 9 in, 2 out]
                            }
                            frame #1 {
                              # "2. 删除框组中指定元素"
                              n178 = local read "部位信息"() -> (w290:string[])
                              n179 = local read "框组"() -> (w292:T3)
                              n180 = Decrement(x=w293) -> (x-1=w289:dbl)
                              n181 = Delete From Array(array=w290, index=w289) -> (array with subset deleted=w288:string[])  [unwired: 1 in, 1 out]
                              n182 = Delete From Array(array=w292, index=w289) -> (array with subset deleted=w291:T3)  [unwired: 1 in, 1 out]
                              n183 = local write "框组"(w291) -> ()
                              n184 = local write "部位信息"(w288) -> ()
                            }
                            frame #2 {
                              # "3. 重画所有框"
                              n185 = while {
                                i -> [w306]
                                stop <- w297 stop-if-true
                                n186 = local read "框组"() -> (w301:T3)
                                n187 = local read "穿透图"() -> (w305:T1)
                                n188 = Array Size(array=w301) -> (size(s)=w302:i32)
                                n189 = Index Array(array=w301, index=w306) -> (element=w296:T17)
                                n190 = Increment(x=w306) -> (x+1=w313:i32)
                                n191 = local write "框数"(w302) -> ()
                                n192 = Greater Or Equal?(x=w313, y=w302) -> (x >= y?=w297:bool)
                                n193 = call "IMAQ Overlay ROI"("ROI Descriptor"=w296, "Image"=w305) -> ("Image Out"=w311:T1)  [unwired: 8 in, 1 out]
                                n194 = Unbundle(w296) -> ("Global Rectangle"=w303:i32[])  [unwired: 1 out]
                                n195 = Number To Decimal String(number=w313) -> (decimal integer string=w298:string)  [unwired: 1 in]
                                n196 = Index Array(array=w303, index=0 ("索引")) -> (element=w308:i32)
                                n197 = Index Array(array=w303, index=1 ("索引")) -> (element=w309:i32)
                                n198 = local read "自定义字体"() -> (w295:T2)
                                n199 = Concatenate Strings(w298, "#" ("字符串")) -> (w294:string)
                                n200 = Bundle(w308, w309) -> (w299:cluster{i32, i32})  [unwired: 1 in]
                                n201 = call "IMAQ Overlay Text"("Text Color (black)"=u32 16711680, "Font, Size & Style"=w295, "String"=w294, "Origin"=w299, "Image"=w311) -> ("Image Out"=w304:T1)  [unwired: 5 in, 1 out]
                                n202 = local write "穿透图"(w304) -> ()
                              }
                            }
                          }
                        }
                      }
                    }
                  }
                  n203 = Wait (ms)(milliseconds to wait=u32 50) -> ()  [unwired: 1 out]
                }
                frame True {
                  n204 = case shown="\"overlay rectangle\"" w317 {
                    tunnel: w319 -> [w331]
                    tunnel: [w330] -> w318
                    tunnel: w316 -> [w329]
                    tunnel: [w328] -> w315
                    tunnel: w314 -> [w320]
                    frame "overlay rectangle" {
                      n205 = flat-sequence {
                        tunnel: w331 -> [w332]
                        tunnel: [w332] -> w327
                        tunnel: w320 -> [w335]
                        tunnel: [w335] -> w326
                        tunnel: w329 -> [w334]
                        tunnel: [w333] -> w325
                        tunnel: w327 -> [w344]
                        tunnel: w326 -> [w343]
                        tunnel: w325 -> [w342]
                        tunnel: [w346] -> w324
                        tunnel: [w342] -> w323
                        tunnel: [w339] -> w322
                        tunnel: [w337] -> w321
                        tunnel: w324 -> [w369]
                        tunnel: w323 -> [w368]
                        tunnel: w322 -> [w360]
                        tunnel: w321 -> [w357]
                        tunnel: [w369] -> w330
                        tunnel: [w368] -> w328
                        frame #0 {
                          # "将当前ROI数据存入框组内"
                          n206 = Build Array (concatenate)(w334, w335) -> (w333:T3)
                          n207 = local write "框组"(w333) -> ()
                        }
                        frame #1 {
                          # "在穿透图上画框"
                          # "图层名Group与“框&图层计数”变量同名，\neg：1号框对应group1"
                          # "overlay text在ROI的左上角添加计数显示"
                          # "overlay ROI代表用户手画绿色框的图层添加"
                          n208 = local read "框组"() -> (w349:T3)
                          n209 = Unbundle(w343) -> ("Global Rectangle"=w352:i32[])  [unwired: 1 out]
                          n210 = Array Size(array=w349) -> (size(s)=w337:i32)
                          n211 = Number To Decimal String(number=w337) -> (decimal integer string=w338:string)  [unwired: 1 in]
                          n212 = local write "框数"(w337) -> ()
                          n213 = Index Array(array=w352, index=1 ("索引")) -> (element=w350:i32)
                          n214 = Index Array(array=w352, index=0 ("索引")) -> (element=w351:i32)
                          n215 = Concatenate Strings(w338, "#" ("字符串")) -> (w339:string)
                          n216 = call "IMAQ Overlay ROI"("Group"=w339, "ROI Descriptor"=w343, "Image"=w344) -> ("Image Out"=w353:T1)  [unwired: 7 in, 1 out]
                          n217 = Bundle(w351, w350) -> (w345:cluster{i32, i32})  [unwired: 1 in]
                          n218 = local read "自定义字体"() -> (w341:T2)
                          n219 = call "IMAQ Overlay Text"("Group"=w339, "Text Color (black)"=u32 16711680, "Font, Size & Style"=w341, "String"=w339, "Origin"=w345, "Image"=w353) -> ("Image Out"=w346:T1)  [unwired: 4 in, 1 out]
                        }
                        frame #2 {
                          # "存放部位信息的1D数组，后续生成报告使用"
                          # "0：位于蒙皮部位\n1：位于筋条部位"
                          n220 = call "缺陷部位标注2"() -> ("位于筋条处"=w365:bool, "位于蒙皮处"=w364:bool)  [unwired: 16 in, 2 out]
                          n221 = Build Array(w364, w365) -> (w366:bool[])
                          n222 = Boolean Array To Number(Boolean array=w366) -> (number=w367:u32)
                          n223 = case shown="1, 默认" w367 {
                            tunnel: ["蒙皮处" ("t") "筋条处" ("t")] -> w355
                            frame 1, Default {
                            }
                            frame 2 {
                            }
                          }
                          n224 = local read "部位信息"() -> (w359:string[])
                          n225 = Decrement(x=w357) -> (x-1=w356:i32)
                          n226 = Insert Into Array(array=w359, index=w356, new element=w355) -> (w358:string[])
                          n227 = Concatenate Strings("框号为" ("字符串"), w360, "\n", "类别为" ("字符串"), w355) -> (w354:string)
                          n228 = local write "连接的字符串"(w354) -> ()
                          n229 = local write "部位信息"(w358) -> ()
                        }
                      }
                    }
                  }
                }
              }
              n230 = local read "完成标注"() -> (w259:bool)
              n231 = case shown="假" w259 {
                tunnel: [FALSE ("T button?") w269] -> w257
                frame False {
                }
                frame True {
                  n232 = Two Button Dialog(message="请确认是否完成标注" ("消息")) -> (T button?=w269:bool)  [unwired: 2 in]
                }
              }
              n233 = local write "穿透图"(w263) -> ()
              n234 = local read "stop"() -> (w262:bool)
              n235 = Or(x=w262, y=w257) -> (x .or. y?=w256:bool)
              n236 = call <vilib>:"Application Directory.vi"() -> ()  [unwired: 1 out]
            }
          }
          frame 1 {
            # "对穿透图和反射图同时画框的分支"
            n237 = while {
              shift-right: [w385] -> _
              shift-left: _ -> [w384]
              tunnel: [w382] -> _
              tunnel: [w381] -> _
              stop <- w375 stop-if-true
              (unwired) "_" ("名称或相对路径")
              (unwired) ".docx" ("名称或相对路径")
              w380 = i32[] [2] items=["No Event"=0, "Click Event"=1, "Draw Event"=2, "Size Event"=4, "Scroll Event"=5, "Double Click Event"=8] ("Which Events")
              # "循环的方式给输入图像手动画框"
              n238 = local read "反射图"() -> (w383:T1)
              n239 = local read "穿透图"() -> (w376:T1)
              n240 = invoke on="穿透图" class="ImageControl" method="Get Last Event"("Which Events"=w380) -> ("Type"=w379:i32)  [unwired: 7 in, 7 out]
              n241 = Not Equal To 0?(x=w379) -> (x != 0?=w386:bool)
              n242 = case shown="假" w386 {
                tunnel: w376 -> [w438 w446]
                tunnel: [w438 w445] -> w382
                tunnel: "Operation" -> [_ w444]
                tunnel: [w437 w439] -> w385
                tunnel: w384 -> [w437 w443]
                tunnel: w383 -> [w436 w442]
                tunnel: [w436 w441] -> w381
                frame False {
                  n243 = Wait (ms)(milliseconds to wait=u32 50 ("毫秒倍数")) -> ()  [unwired: 1 out]
                }
                frame True {
                  n244 = property on="穿透图" class="ImageControl"() -> ("ROI"=w440:T17)  [unwired: 2 in, 2 out]
                  n245 = case shown="\"overlay rectangle\"" w444 {
                    tunnel: w446 -> [w462]
                    tunnel: w440 -> [w460]
                    tunnel: [w461] -> w445
                    tunnel: w443 -> [w459]
                    tunnel: w442 -> [w458]
                    tunnel: [w457] -> w441
                    tunnel: [w456] -> w439
                    frame "overlay rectangle" {
                      n246 = flat-sequence {
                        tunnel: w462 -> [w465]
                        tunnel: [w465] -> w455
                        tunnel: w460 -> [w467]
                        tunnel: [w467] -> w454
                        tunnel: w459 -> [w466]
                        tunnel: w458 -> [w464]
                        tunnel: [w464] -> w453
                        tunnel: [w463] -> w452
                        tunnel: w455 -> [w476]
                        tunnel: w454 -> [w475]
                        tunnel: w453 -> [w481]
                        tunnel: w452 -> [w473]
                        tunnel: [w482] -> w451
                        tunnel: [w480] -> w450
                        tunnel: [w473] -> w449
                        tunnel: [w471] -> w448
                        tunnel: [w469] -> w447
                        tunnel: w451 -> [w506]
                        tunnel: w450 -> [w505]
                        tunnel: w449 -> [w504]
                        tunnel: w448 -> [w495]
                        tunnel: w447 -> [w492]
                        tunnel: [w506] -> w461
                        tunnel: [w505] -> w457
                        tunnel: [w504] -> w456
                        frame #0 {
                          # "将当前ROI数据存入框组内"
                          n247 = Build Array (concatenate)(w466, w467) -> (w463:T3)
                          n248 = local write "框组"(w463) -> ()
                        }
                        frame #1 {
                          w478 = u32[] [15663114] ("Colors (Green)")
                          w474 = u32 16711776 ("Text Color (black)")
                          # "在反射图上对应位置画框"
                          # "在穿透图上画框"
                          # "图层名Group与“框&图层计数”变量同名，\neg：1号框对应group1"
                          # "overlay text在ROI的左上角添加计数显示"
                          # "overlay ROI代表用户手画绿色框的图层添加"
                          n249 = local read "框组"() -> (w485:T3)
                          n250 = Array Size(array=w485) -> (size(s)=w469:i32)
                          n251 = Unbundle(w475) -> ("Global Rectangle"=w488:i32[])  [unwired: 1 out]
                          n252 = Number To Decimal String(number=w469) -> (decimal integer string=w470:string)  [unwired: 1 in]
                          n253 = local write "框数"(w469) -> ()
                          n254 = Concatenate Strings(w470, "#" ("字符串")) -> (w471:string)
                          n255 = Index Array(array=w488, index=1 ("索引")) -> (element=w486:i32)
                          n256 = Index Array(array=w488, index=0 ("索引")) -> (element=w487:i32)
                          n257 = local read "自定义字体"() -> (w472:T2)
                          n258 = call "IMAQ Overlay ROI"("Colors (Green)"=w478, "Group"=w471, "ROI Descriptor"=w475, "Image"=w476) -> ("Image Out"=w489:T1)  [unwired: 6 in, 1 out]
                          n259 = call "IMAQ Overlay ROI"("Colors (Green)"=w478, "Group"=w471, "ROI Descriptor"=w475, "Image"=w481) -> ("Image Out"=w479:T1)  [unwired: 6 in, 1 out]
                          n260 = Bundle(w487, w486) -> (w477:cluster{i32, i32})  [unwired: 1 in]
                          n261 = call "IMAQ Overlay Text"("Group"=w471, "Text Color (black)"=w474, "Font, Size & Style"=w472, "String"=w471, "Origin"=w477, "Image"=w479) -> ("Image Out"=w480:T1)  [unwired: 4 in, 1 out]
                          n262 = call "IMAQ Overlay Text"("Group"=w471, "Text Color (black)"=w474, "Font, Size & Style"=w472, "String"=w471, "Origin"=w477, "Image"=w489) -> ("Image Out"=w482:T1)  [unwired: 4 in, 1 out]
                        }
                        frame #2 {
                          # "存放部位信息的1D数组，后续生成报告使用"
                          # "0：位于蒙皮部位\n1：位于筋条部位"
                          n263 = call "缺陷部位标注"() -> ("位于筋条处"=w500:bool, "位于蒙皮处"=w499:bool)  [unwired: 16 in, 2 out]
                          n264 = Build Array(w499, w500) -> (w501:bool[])
                          n265 = Boolean Array To Number(Boolean array=w501) -> (number=w502:u32)
                          n266 = local read "部位信息"() -> (w494:string[])
                          n267 = case shown="1, 默认" w502 {
                            tunnel: ["蒙皮处" ("t") "筋条处" ("t")] -> w490
                            frame 1, Default {
                            }
                            frame 2 {
                            }
                          }
                          n268 = Decrement(x=w492) -> (x-1=w491:i32)
                          n269 = Insert Into Array(array=w494, index=w491, new element=w490) -> (w493:string[])
                          n270 = Concatenate Strings("框号为" ("字符串"), w495, "\n", "类别为" ("字符串"), w490) -> (→"连接的字符串":string)
                          n271 = local write "部位信息"(w493) -> ()
                        }
                      }
                    }
                  }
                }
              }
              n272 = event shown="[1] \"查看标注\": 鼠标按下" {
                selector: _ -> [_ _]
                dyn-events: _ -> [_ _]
                timeout: 50 -> [_ _]
                event Timeout {
                  n273 = event-data() -> ()  [unwired: 1 in, 3 out]
                }
                event "查看标注": Mouse Down {
                  n274 = event-data() -> ()  [unwired: 1 in, 8 out]
                  n275 = local read "反射图原始路径"() -> (w427:path)
                  n276 = local read "穿透图原始路径"() -> (w428:path)
                  n277 = local read "临界面积百分比值"() -> (w424:dbl)
                  n278 = local read "部位信息"() -> (w430:string[])
                  n279 = local read "产品规格"() -> (w429:cluster{"产品长度（周长）（mm）":dbl, "产品宽度（母线长）（mm）":dbl})
                  n280 = local read "框组"() -> (w425:T3)
                  n281 = local read "临界Z值"() -> (w426:i32)
                  n282 = local read "灰度阈值"() -> (w423:dbl)
                  n283 = call "输入选择框号"() -> ("框号"=w431:dbl)  [unwired: 17 in, 2 out]
                  n284 = call "子界面-查看某框.vi"("框号"=w431, "框组"=w425, "临界Z值"=w426, "反射图原始路径"=w427, "临界面积百分比值"=w424, "预先配置的灰度阈值"=w423, "穿透图原始路径"=w428, "部位信息"=w430, "产品规格"=w429) -> ()  [unwired: 9 in, 2 out]
                }
              }
              n285 = event shown="[1] \"删除标注\": 鼠标按下" {
                selector: _ -> [_ _]
                dyn-events: _ -> [_ _]
                timeout: 50 -> [_ _]
                event Timeout {
                  n286 = event-data() -> ()  [unwired: 1 in, 3 out]
                }
                event "删除标注": Mouse Down {
                  n287 = event-data() -> ()  [unwired: 1 in, 3 out]
                  n288 = call "用户输入"() -> ("框号"=w389:dbl, "确定"=w388:bool)  [unwired: 17 in, 1 out]
                  n289 = case shown="真" w388 {
                    tunnel: w389 -> [_ w390]
                    frame False {
                      # "用户取消操作"
                    }
                    frame True {
                      n290 = stacked-sequence {
                        tunnel: w390 -> [_ w393 _]
                        frame #0 {
                          # "1. 删除所有框"
                          n291 = local read "穿透图"() -> (w391:T1)
                          n292 = local read "反射图"() -> (w392:T1)
                          n293 = call "IMAQ Clear Overlay"("Image"=w392) -> ()  [unwired: 9 in, 2 out]
                          n294 = call "IMAQ Clear Overlay"("Image"=w391) -> ()  [unwired: 9 in, 2 out]
                        }
                        frame #1 {
                          # "2. 删除框组中指定元素"
                          n295 = local read "部位信息"() -> (w396:string[])
                          n296 = local read "框组"() -> (w398:T3)
                          n297 = Decrement(x=w393) -> (x-1=w395:dbl)
                          n298 = Delete From Array(array=w398, index=w395) -> (array with subset deleted=w397:T3)  [unwired: 1 in, 1 out]
                          n299 = Delete From Array(array=w396, index=w395) -> (array with subset deleted=w394:string[])  [unwired: 1 in, 1 out]
                          n300 = local write "框组"(w397) -> ()
                          n301 = local write "部位信息"(w394) -> ()
                        }
                        frame #2 {
                          # "3. 重画所有框"
                          n302 = while {
                            i -> [w413]
                            stop <- w402 stop-if-true
                            n303 = local read "框组"() -> (w406:T3)
                            n304 = local read "反射图"() -> (w407:T1)
                            n305 = local read "穿透图"() -> (w412:T1)
                            n306 = Array Size(array=w406) -> (size(s)=w409:i32)
                            n307 = Index Array(array=w406, index=w413) -> (element=w401:T17)
                            n308 = Increment(x=w413) -> (x+1=w422:i32)
                            n309 = local write "框数"(w409) -> ()
                            n310 = Greater Or Equal?(x=w422, y=w409) -> (x >= y?=w402:bool)
                            n311 = call "IMAQ Overlay ROI"("ROI Descriptor"=w401, "Image"=w407) -> ("Image Out"=w415:T1)  [unwired: 8 in, 1 out]
                            n312 = call "IMAQ Overlay ROI"("ROI Descriptor"=w401, "Image"=w412) -> ("Image Out"=w420:T1)  [unwired: 8 in, 1 out]
                            n313 = Unbundle(w401) -> ("Global Rectangle"=w410:i32[])  [unwired: 1 out]
                            n314 = Number To Decimal String(number=w422) -> (decimal integer string=w403:string)  [unwired: 1 in]
                            n315 = Index Array(array=w410, index=0 ("索引")) -> (element=w417:i32)
                            n316 = Index Array(array=w410, index=1 ("索引")) -> (element=w418:i32)
                            n317 = local read "自定义字体"() -> (w400:T2)
                            n318 = Concatenate Strings(w403, "#" ("字符串")) -> (w399:string)
                            n319 = Bundle(w417, w418) -> (w404:cluster{i32, i32})  [unwired: 1 in]
                            n320 = call "IMAQ Overlay Text"("Text Color (black)"=u32 16711680, "Font, Size & Style"=w400, "String"=w399, "Origin"=w404, "Image"=w415) -> ("Image Out"=w408:T1)  [unwired: 5 in, 1 out]
                            n321 = call "IMAQ Overlay Text"("Text Color (black)"=u32 16711680, "Font, Size & Style"=w400, "String"=w399, "Origin"=w404, "Image"=w420) -> ("Image Out"=w411:T1)  [unwired: 5 in, 1 out]
                            n322 = local write "反射图"(w408) -> ()
                            n323 = local write "穿透图"(w411) -> ()
                          }
                        }
                      }
                    }
                  }
                }
              }
              n324 = case shown="真" "完成标注" {
                tunnel: [FALSE ("T button?") w434] -> w372
                frame False {
                }
                frame True {
                  n325 = Two Button Dialog(message="请确认是否完成标注" ("消息")) -> (T button?=w434:bool)  [unwired: 2 in]
                }
              }
              n326 = local write "穿透图"(w382) -> ()
              n327 = local write "反射图"(w381) -> ()
              n328 = local read "stop"() -> (w378:bool)
              n329 = Or(x=w378, y=w372) -> (x .or. y?=w375:bool)
              n330 = call <vilib>:"Application Directory.vi"() -> ()  [unwired: 1 out]
            }
          }
        }
      }
      event "查看标注": Value Change {
        # "查看指定框的详细信息，包括灰度和面积阈值分割后的结果，提取到的长宽面积等信息"
        n331 = event-data() -> ()  [unwired: 1 in, 6 out]
        n332 = local read "模式选择"() -> (w520:u16)
        n333 = local read "临界面积百分比值"() -> (w512:dbl)
        n334 = local read "穿透图原始路径"() -> (w517:path)
        n335 = local read "临界Z值"() -> (w513:i32)
        n336 = local read "灰度阈值"() -> (w509:dbl)
        n337 = local read "部位信息"() -> (w519:string[])
        n338 = local read "产品规格"() -> (w518:cluster{"产品长度（周长）（mm）":dbl, "产品宽度（母线长）（mm）":dbl})
        n339 = local read "框组"() -> (w514:T3)
        n340 = call "输入选择框号"() -> ("框号"=w516:dbl, "确定"=w515:bool)  [unwired: 17 in, 1 out]
        n341 = case shown="1" w520 {
          tunnel: w519 -> [w530 w554]
          tunnel: w518 -> [w529 w553]
          tunnel: w517 -> [w528 w552]
          tunnel: w516 -> [w527 w551]
          tunnel: w515 -> [w531 w550]
          tunnel: w514 -> [w526 w549]
          tunnel: w513 -> [w525 w548]
          tunnel: w512 -> [w524 w547]
          tunnel: [w521 w546] -> w511
          tunnel: [w522 w545] -> w510
          tunnel: w509 -> [w523 w544]
          frame 0, Default {
            # "只读穿透图的图像处理方法"
            n342 = case shown="真" w531 {
              tunnel: w530 -> [_ w543]
              tunnel: w529 -> [_ w542]
              tunnel: w528 -> [_ w534]
              tunnel: w527 -> [_ w541]
              tunnel: w526 -> [_ w540]
              tunnel: w525 -> [_ w539]
              tunnel: w524 -> [_ w538]
              tunnel: w523 -> [_ w537]
              tunnel: [w533 w536] -> w522
              tunnel: [w532 w535] -> w521
              frame False {
                n343 = local read "分层类检测结果"() -> (w533:string[][])
                n344 = local read "弥散类检测结果"() -> (w532:string[][])
              }
              frame True {
                n345 = call "子界面-查看某框-只读穿透图模式.vi"("框号"=w541, "框组"=w540, "临界Z值"=w539, "临界面积百分比值"=w538, "预先配置的灰度阈值"=w537, "穿透图原始路径"=w534, "部位信息"=w543, "产品规格"=w542) -> ("弥散类检测结果"=w535:string[][], "分层类检测结果"=w536:string[][])  [unwired: 10 in]
              }
            }
          }
          frame 1 {
            # "穿透图和反射图结合的图像处理方法"
            n346 = local read "反射图原始路径"() -> (w555:path)
            n347 = case shown="真" w550 {
              tunnel: w551 -> [_ w568]
              tunnel: w544 -> [_ w567]
              tunnel: w553 -> [_ w566]
              tunnel: w554 -> [_ w565]
              tunnel: w552 -> [_ w559]
              tunnel: w555 -> [_ w558]
              tunnel: w549 -> [_ w564]
              tunnel: w548 -> [_ w563]
              tunnel: w547 -> [_ w562]
              tunnel: [w556 w561] -> w546
              tunnel: [w557 w560] -> w545
              frame False {
                # "用户取消操作"
                n348 = local read "弥散类检测结果"() -> (w556:string[][])
                n349 = local read "分层类检测结果"() -> (w557:string[][])
              }
              frame True {
                n350 = call "子界面-查看某框.vi"("框号"=w568, "框组"=w564, "临界Z值"=w563, "反射图原始路径"=w558, "临界面积百分比值"=w562, "预先配置的灰度阈值"=w567, "穿透图原始路径"=w559, "部位信息"=w565, "产品规格"=w566) -> ("弥散类检测结果"=w561:string[][], "分层类检测结果"=w560:string[][])  [unwired: 9 in]
              }
            }
          }
        }
        "弥散类检测结果" <- w511
        "分层类检测结果" <- w510
      }
      event "生成评定结果": Value Change {
        # "最终检测结果全部合并 导入word中"
        # "相当于“查看标注”一栏中的操作做循环，遍历所有框，\n将输出结果叠加为数组，作为最终结果输出并导入word"
        n351 = event-data() -> ()  [unwired: 1 in, 6 out]
        n352 = local read "分层类检测结果合并"() -> (w582:string[][])
        n353 = local read "弥散类检测结果合并"() -> (w580:string[][])
        n354 = local read "模式选择"() -> (w590:u16)
        n355 = local read "临界面积百分比值"() -> (w583:dbl)
        n356 = local read "穿透图原始路径"() -> (w587:path)
        n357 = local read "灰度阈值"() -> (w581:dbl)
        n358 = local read "临界Z值"() -> (w584:i32)
        n359 = local read "部位信息"() -> (w589:string[])
        n360 = local read "产品规格"() -> (w588:cluster{"产品长度（周长）（mm）":dbl, "产品宽度（母线长）（mm）":dbl})
        n361 = local read "框组"() -> (w586:T3)
        n362 = local read "框数"() -> (w585:dbl)
        n363 = case shown="1" w590 {
          tunnel: [w599 w634] -> w594
          tunnel: [w597 w624] -> w593
          tunnel: w589 -> [w607 w633]
          tunnel: w588 -> [w605 w632]
          tunnel: w587 -> [w604 w631]
          tunnel: w586 -> [w603 w630]
          tunnel: w585 -> [w606 w629]
          tunnel: w581 -> [_ w628]
          tunnel: w584 -> [w602 w627]
          tunnel: w583 -> [w601 w626]
          tunnel: w582 -> [w598 w625]
          tunnel: w581 -> [w600 _]
          tunnel: w580 -> [w596 w623]
          frame 0, Default {
            # "只读穿透图的图像处理方法"
            n364 = for {
              N: w606 -> [_]
              tunnel: w607 -> [w622]
              tunnel: w605 -> [w621]
              tunnel: w604 -> [w608]
              tunnel: w603 -> [w620]
              tunnel: w602 -> [w619]
              tunnel: w601 -> [w618]
              tunnel: w600 -> [w617]
              shift-right: [w615] -> w599
              shift-left: w598 -> [w614]
              shift-right: [w609] -> w597
              shift-left: w596 -> [w610]
              i -> [w613]
              n365 = Increment(x=w613) -> (x+1=w612:i32)
              n366 = call "子界面-查看某框-不显示界面-只读穿透图模式.vi"("框号"=w612, "框组"=w620, "临界Z值"=w619, "临界面积百分比值"=w618, "预先配置的灰度阈值"=w617, "穿透图原始路径"=w608, "部位信息"=w622, "产品规格"=w621) -> ("弥散类检测结果"=w611:string[][], "分层类检测结果"=w616:string[][])  [unwired: 10 in]
              n367 = Build Array (concatenate)(w610, w611) -> (w609:string[][])
              n368 = Build Array (concatenate)(w614, w616) -> (w615:string[][])
            }
          }
          frame 1 {
            # "穿透图和反射图结合的图像处理方法"
            n369 = local read "反射图原始路径"() -> (w635:path)
            n370 = for {
              N: w629 -> [_]
              tunnel: w635 -> [w636]
              shift-right: [w641] -> w634
              shift-left: w625 -> [w643]
              tunnel: w633 -> [w651]
              tunnel: w632 -> [w650]
              tunnel: w631 -> [w637]
              tunnel: w630 -> [w649]
              tunnel: w628 -> [w648]
              tunnel: w627 -> [w647]
              tunnel: w626 -> [w646]
              shift-right: [w640] -> w624
              shift-left: w623 -> [w638]
              i -> [w645]
              n371 = Increment(x=w645) -> (x+1=w644:i32)
              n372 = call "子界面-查看某框-不显示界面.vi"("框号"=w644, "框组"=w649, "临界Z值"=w647, "反射图原始路径"=w636, "临界面积百分比值"=w646, "预先配置的灰度阈值"=w648, "穿透图原始路径"=w637, "部位信息"=w651, "产品规格"=w650) -> ("弥散类检测结果"=w639:string[][], "分层类检测结果"=w642:string[][])  [unwired: 9 in]
              n373 = Build Array (concatenate)(w643, w642) -> (w641:string[][])
              n374 = Build Array (concatenate)(w638, w639) -> (w640:string[][])
            }
          }
        }
        n375 = local write "弥散类检测结果合并"(w593) -> ()
        n376 = local write "分层类检测结果合并"(w594) -> ()
        n377 = flat-sequence {
          tunnel: w593 -> [w652]
          tunnel: w594 -> [w653]
          tunnel: [w653] -> w572
          tunnel: [w652] -> w570
          tunnel: w572 -> [w694]
          tunnel: [w694] -> w571
          tunnel: w570 -> [w693]
          tunnel: [w693] -> w569
          tunnel: w571 -> [w701]
          tunnel: w569 -> [w700]
          tunnel: [w701] -> w579
          tunnel: [w700] -> w578
          tunnel: [w699] -> w576
          tunnel: [w698] -> w575
          tunnel: [w721] -> w592
          tunnel: [w720] -> w591
          tunnel: w579 -> [w711]
          tunnel: w578 -> [w714]
          tunnel: [w714] -> w577
          tunnel: w576 -> [w713]
          tunnel: w575 -> [w712]
          tunnel: w592 -> [w732]
          tunnel: w591 -> [w731]
          tunnel: w577 -> [w730]
          tunnel: [w729] -> w574
          tunnel: [w728] -> w573
          tunnel: w574 -> [w748]
          tunnel: w573 -> [w747]
          frame #0 {
            n378 = while {
              tunnel: [w660] -> _
              i -> [w664]
              stop <- w660 stop-if-true
              w669 = 1 items=["White", "Black", "Inverted", "Black on White", "White on Black"] ("Color")
              w673 = u16 2 items=["Frame", "Paint", "Invert Frame", "Invert Paint"] ("Draw Mode")
              w666 = u16 1 items=["Line", "Rectangle", "Oval"] ("Shape to draw")
              # "生成绘制了ROI的图像\n可以用于后续的图片导出保存"
              n379 = local read "框组"() -> (w663:T3)
              n380 = local read "穿透图"() -> (w656:T1)
              n381 = Array Size(array=w663) -> (size(s)=w681:i32)
              n382 = local read "ROImask"() -> (w655:T1)
              n383 = Index Array(array=w663, index=w664) -> (element=w662:T17)
              n384 = Unbundle(w662) -> ("Global Rectangle"=w661:i32[])  [unwired: 1 out]
              n385 = Increment(x=w664) -> (x+1=w682:i32)
              n386 = Greater Or Equal?(x=w682, y=w681) -> (x >= y?=w660:bool)
              n387 = Index Array(array=w661, index=0 ("索引")) -> (element=w671:i32)
              n388 = Index Array(array=w661, index=2 ("索引")) -> (element=w676:i32)
              n389 = Index Array(array=w661, index=1 ("索引")) -> (element=w670:i32)
              n390 = Index Array(array=w661, index=3 ("索引")) -> (element=w675:i32)
              n391 = Number To Decimal String(number=w682) -> (decimal integer string=w667:string)  [unwired: 1 in]
              n392 = Build Array(w671, w670, w676, w675) -> (w657:i32[])
              n393 = call "IMAQ Draw"("Draw Mode"=w673, "Shape to draw"=w666, "Pixel Color"=sgl 0.0, "Coordinates"=w657, "Image Src"=w656) -> ("Image Dst Out"=w672:T1)  [unwired: 5 in, 1 out]
              n394 = Concatenate Strings(w667, "#" ("字符串")) -> (w665:string)
              n395 = local read "自定义字体"() -> (w658:T2)
              n396 = Build Array(w671, w670) -> (w659:i32[])
              n397 = call "IMAQ Draw Text"("String"=w665, "Insertion Point"=w659, "Color"=w669, "Font, Size & Style"=w658, "Image Dst"=w655, "Image Src"=w672) -> ("Image Dst Out"=w654:T1)  [unwired: 2 in, 3 out]
              "ROImask" <- w654
              n398 = local write "ROImask"(w654) -> ()
            }
          }
          frame #1 {
            n399 = local read "穿透图原始路径"() -> (w692:path)
            n400 = local read "ROImask"() -> (w683:T1)
            n401 = Path To String(path=w692) -> (string=w689:string)
            n402 = String Length(string=w689) -> (length=w690:i32)
            n403 = Subtract(x=w690, y=4) -> (x-y=w691:i32)
            n404 = Replace Substring(3:w691, 4:"_标注后.png" ("字符串"), 5:w689) -> (1:w688:string)  [unwired: 1 in, 1 out]
            n405 = String To Path(string=w688) -> (path=w684:path)
            "标注后的图片路径" <- w684
            n406 = call-poly "IMAQ Write File 2"("Image Quality"=u32 1000, "File Path"=w684, "Image"=w683) -> ()  [unwired: 7 in, 2 out]
          }
          frame #2 {
            n407 = call <vilib>:"Application Directory.vi"() -> ("Application Directory"=w697:path)
            n408 = Build Path(base path=w697, name or relative path="report-template.docx") -> (appended path=w695:path)
            n409 = call <vilib>:"Create Report.vi"("window state (normal)"=T9."maximized", "report type"=Report_Type."Word", "template (empty)"=w695) -> ("report out"=w699:refnum<class "NI_report.lvclass">, "error out"=w698:errorcluster)  [unwired: 11 in]
          }
          frame #3 {
            n410 = Get Date/Time String(date format (0)=enum16{"short", "long", "abbreviated"}."long" ("日期格式(0)")) -> (date string=w718:string, time string=w719:string)  [unwired: 2 in]
            n411 = local read "标注后的图片路径"() -> (w709:path)
            n412 = Concatenate Strings(w718, w719) -> (w717:string)
            n413 = call-poly <vilib>:"Append Report Text.vi"("report in"=w713, "MS Office parameters"=T13 {"position (excel)"={"row"=0, "column"=0}, "name (excel)"="", "bookmark (word)"="time"}, "text"=w717, "error in (no error)"=w712) -> ("report out"=w708:refnum<class "NI_report.lvclass">, "error out"=w706:errorcluster)  [unwired: 8 in, 2 out]
            n414 = call-poly <vilib>:"Append Image to Report.vi"("report in"=w708, "alignment (default)"=HTML_Report_Image_Alignment."MIDDLE", "MS Office parameters"=T12 {"position (Excel)"={"row"=0, "column"=0}, "name (Excel)"="", "bookmark (Word)"="image"}, "path or URL of image"=w709, "error in (no error)"=w706) -> ("report out"=w705:refnum<class "NI_report.lvclass">, "error out"=w704:errorcluster)  [unwired: 7 in, 2 out]
            n415 = call <vilib>:"Word Easy Text.vi"("report in"=w705, "text"="分层类", "alignment (left)"=enum16{"Left", "Centered", "Right", "Justify"}."Left", "font"=T14 {"font name"="", "font size"=0.0, "bold"=0, "italic"=0, "underline"=0, "strike through"=0, "font color"=16777216}, "error in (no error)"=w704) -> ("report out"=w723:refnum<class "NI_report.lvclass">, "error out"=w724:errorcluster)  [unwired: 8 in, 1 out]
            n416 = call-poly <vilib>:"Word Easy Table.vi"("report in"=w723, "column headers"=string[] ["框号", "长/mm", "宽/mm", "面积/mm2", "Z值/mm", "部位", "类型", "合格性"], "data"=w711, "error in (no error)"=w724) -> ("report out"=w721:refnum<class "NI_report.lvclass">, "error out"=w720:errorcluster)  [unwired: 9 in, 1 out]
          }
          frame #4 {
            n417 = call <vilib>:"Word Easy Text.vi"("report in"=w732, "text"="弥散类", "alignment (left)"=enum16{"Left", "Centered", "Right", "Justify"}."Left", "font"=T14 {"font name"="", "font size"=0.0, "bold"=0, "italic"=0, "underline"=0, "strike through"=0, "font color"=16777216}, "error in (no error)"=w731) -> ("report out"=w734:refnum<class "NI_report.lvclass">, "error out"=w735:errorcluster)  [unwired: 8 in, 1 out]
            n418 = call-poly <vilib>:"Word Easy Table.vi"("report in"=w734, "column headers"=string[] ["框号", "长/mm", "宽/mm", "面积/mm2", "Z值/mm", "部位", "类型", "合格性"], "data"=w730, "error in (no error)"=w735) -> ("report out"=w729:refnum<class "NI_report.lvclass">, "error out"=w728:errorcluster)  [unwired: 9 in, 1 out]
          }
          frame #5 {
            n419 = local read "穿透图原始路径"() -> (w739:path)
            n420 = Path To String(path=w739) -> (string=w744:string)
            n421 = String Length(string=w744) -> (length=w745:i32)
            n422 = Subtract(x=w745, y=4) -> (x-y=w746:i32)
            n423 = Replace Substring(3:w746, 4:"_.docx" ("字符串"), 5:w744) -> (1:w743:string)  [unwired: 1 in, 1 out]
            n424 = String To Path(string=w743) -> (path=w740:path)
            "添加的路径" <- w740
            n425 = call-dynamic "Save Report to File.vi"("report in"=w748, "report file path"=w740, "prompt to replace? (F)"=TRUE, "error in (no error)"=w747) -> ("report out"=w752:refnum<class "NI_report.lvclass">, "error out"=w751:errorcluster)  [unwired: 10 in]
            n426 = call <vilib>:"Word Bring to Front.vi"("report in"=w752, "window state (maximized)"=enum16{"maximized", "minimized", "normal"}."normal", "error in (no error)"=w751) -> ()  [unwired: 11 in, 2 out]
          }
          frame #6 {
            n427 = One Button Dialog(message="完成评定并退出程序！\n请查看word报告" ("消息")) -> ()  [unwired: 1 in, 1 out]
          }
        }
      }
      event "stop": Value Change {
        # "退出软件"
        n428 = event-data() -> ("NewVal"=w757:bool)  [unwired: 1 in, 4 out]
        n429 = Two Button Dialog(message="是否关闭本软件？" ("消息")) -> (T button?=w758:bool)  [unwired: 2 in]
        n430 = And(x=w757, y=w758) -> (x .and. y?=w756:bool)
        n431 = case shown="真" w756 {
          frame False {
          }
          frame True {
            w759 = TRUE ("All Images? (No)")
            n432 = local read "穿透图"() -> (w761:T1)
            n433 = local read "反射图"() -> (w760:T1)
            n434 = call "IMAQ Dispose"("All Images? (No)"=w759, "Image"=w761) -> ()  [unwired: 4 in, 1 out]
            n435 = call "IMAQ Dispose"("All Images? (No)"=w759, "Image"=w760) -> ()  [unwired: 4 in, 1 out]
            n436 = disable-structure shown="RUN_TIME_ENGINE==True" {
              frame condition #0 {
                n437 = Quit LabVIEW() -> ()  [unwired: 1 in]
              }
              frame condition #1 (active) {
                n438 = Stop() -> ()  [unwired: 1 in]
              }
            }
          }
        }
      }
    }
  }
  n439 = disable-structure shown="禁用" {
    frame Disabled {
      n440 = while {
        stop <- FALSE stop-if-true
        n441 = local read "删除标注"() -> (w765:bool)
        n442 = local read "查看标注"() -> (w764:bool)
        n443 = Or(x=w765, y=w764) -> (x .or. y?=w766:bool)
        n444 = local write "开始标注"(w766) -> ()
        n445 = Wait Until Next ms Multiple(millisecond multiple=u32 50 ("毫秒倍数")) -> ()  [unwired: 1 out]
      }
    }
    frame Enabled {
    }
  }
  "框组" <- T3 [] ("框组")
  "框数" <- 0.0 ("框数")
  "自定义字体" <- T2 {"Desired Font (Application)"=enum."User-specified Font", "[User-specified Font]"={"Font Name"="", "Size"=80, "Strikeout?"=FALSE, "Italic?"=FALSE, "Underline?"=FALSE, "Outline?"=FALSE, "Shadow?"=FALSE, "Bold?"=TRUE, "Rotation Angle"=0.0}, "Horizontal Alignment"=0, "Vertical Alignment"=0} ("Font, Size & Style")
  "部位信息" <- string[] ["", "", "", "", "", "", "", "", ""] ("部位信息")
  "分层类检测结果合并" <- string[][] [] ("弥散类检测结果合并")
  "弥散类检测结果合并" <- string[][] [] ("弥散类检测结果合并")
  "临界面积百分比值" <- w4
  "输入的灰度阈值" <- w5
